vi "CSM Dummy Module.vi"(7 "Name (\"\" to Use UUID)":string="JKISM-Module") -> ()   [LabVIEW 2017, in "Communicable State Machine.lvlib"]
doc: "### CSM Dummy Module.vi\n\n-- <b>Controls</b> --\n- <b>Init State(\"Macro: Initialize\")</b>:\n- <b>Name(\"\" to use uuid)</b>:"
uses:
  Communicable State Machine.lvlib
panel:
  # "Replace this dummy moudule with your own CSM Module"
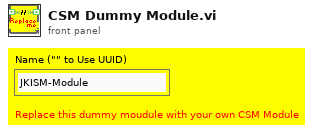
[diagram p1: front panel]
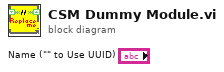
[diagram p0: block diagram]
diagram:
